vi "write odors to spreadhseet.vi"(9 "measurements":T1, 10 "write odors?":bool, 11 "file path":path) -> ()   [LabVIEW 2013]
uses:
  <vilib>/Utility/file.llb/Write To Spreadsheet File (DBL).vi
  <vilib>/Utility/file.llb/Write To Spreadsheet File (string).vi
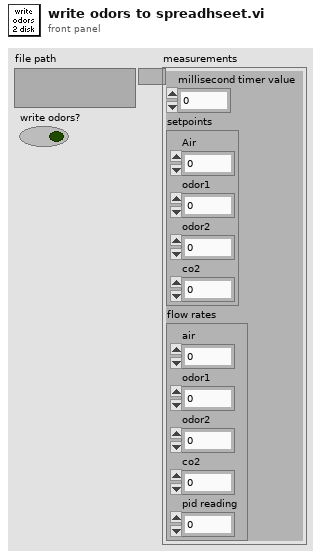
[diagram p1: front panel]
types:
  T1 = cluster{"millisecond timer value":u32, "setpoints ":cluster{"Air ":dbl, "odor1":dbl, "odor2":dbl, "co2":dbl}, "flow rates":cluster{"air":dbl, "odor1":dbl, "odor2":dbl, "co2":dbl, "pid reading":dbl}}
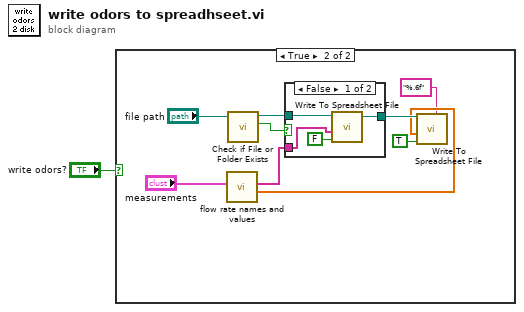
[diagram p0: block diagram]
diagram:
  n1 = case shown="True" "write odors?" {
    frame False {
    }
    frame True {
      n2 = call "flow rate names and values.vi"("measurements"="measurements") -> ("values"=w3:dbl[], "names"=w7:string[])  [unwired: 9 in]
      n3 = call <vilib>:"Check if File or Folder Exists.vi"("path"="file path") -> ("file or folder exists?"=w8:bool, "dup path"=w6:path)  [unwired: 8 in, 1 out]
      n4 = case shown="False" w8 {
        tunnel: w6 -> [w13 w15]
        tunnel: w7 -> [w12 _]
        tunnel: [w11 w15] -> w5
        frame False {
          n5 = call-poly <vilib>:"Write To Spreadsheet File.vi"("append to file? (new file:F)"=FALSE, "1D data"=w12, "file path (dialog if empty)"=w13) -> ("new file path (Not A Path if cancelled)"=w11:path)  [unwired: 5 in]
        }
        frame True {
        }
      }
      n6 = call-poly <vilib>:"Write To Spreadsheet File.vi"("format (%.3f)"="%.6f", "append to file? (new file:F)"=TRUE, "1D data"=w3, "file path (dialog if empty)"=w5) -> ()  [unwired: 4 in, 1 out]
    }
  }
